vi "test_psmc.vi"() -> ()   [LabVIEW 2014]
uses:
  <vilib>/Platform/TimedLoop/XDataNode/timing_clust.ctl
  <vilib>/Platform/TimedLoop/XDataNode/nitl_modes.ctl
  <vilib>/Platform/TimedLoop/XDataNode/wakeup.ctl
  <vilib>/platform/TimedLoop/XDataNode/XDataNode.xnode
  <vilib>/Platform/TimedLoop/XDataNode/XDNodeRunTimeDep.lvlib
  <vilib>/ptbypt/NI_PtbyPt.lvlib
panel:
  in  "pd":dbl
  out "M1":T1(graph)={"M1 desired speed"=-0.04979126824650304, "M1 position"=nan}
  in  "stop":bool
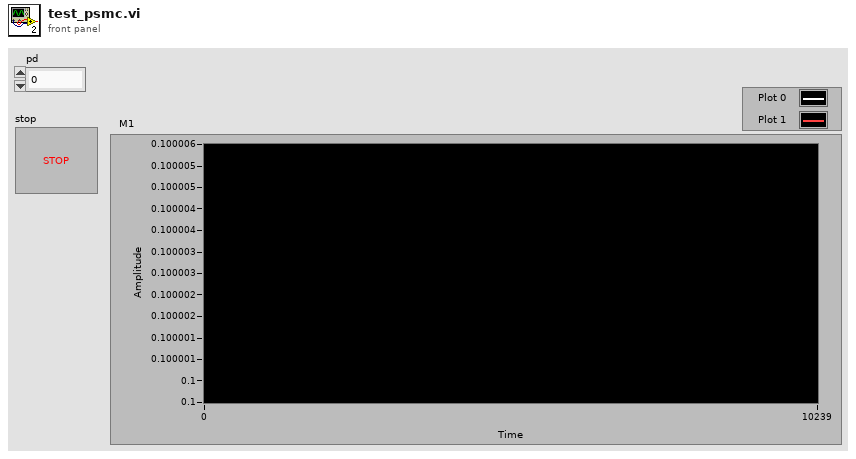
[diagram p1: front panel]
types:
  T1 = cluster{"M1 desired speed":dbl, "M1 position":dbl}
  T2 = typedef "XDNodeRunTimeDep.lvlib/timing_clust.ctl" = cluster{"Expected End [f-1]":u64, "Actual End [f-1]":u64, "Finished Late? [f-1]":bool, "Expected End [i-1]":u64, "Actual End [i-1]":u64, "Finished Late? [i-1]":bool, "Expected Start [i]":u64, "Actual Start [i]":u64, "Expected Start [f]":u64, "Actual Start [f]":u64, "Source Name":string, "Structure Name":string, "Period":i64, "Deadline":i64, "Offset":i64, "Start":i64, "Priority":i32, "Timeout":i32, "Mode":T3, "Wakeup Reason":T4, "Error":errorcluster, "Source Type":string, "Secondary Source Type":string, "Global End Time":u64, "Global Start Time":u64, "Frame Duration":u64, "Iteration Duration":u64, "Assigned CPU":i32, "I/O Scan Engine Mode":u32}
  T3 = typedef "XDNodeRunTimeDep.lvlib/nitl_modes.ctl" = enum32{"No Change", "Process missed periods, maintain original phase", "Discard missed periods, maintain original phase", "Process missed periods, ignore original phase", "Discard missed periods, ignore original phase"}
  T4 = typedef "XDNodeRunTimeDep.lvlib/wakeup.ctl" = enum32{"Normal", "Aborted", "Asynchronous wakeup", "Timing source error", "Timed loop error", "Timeout"}
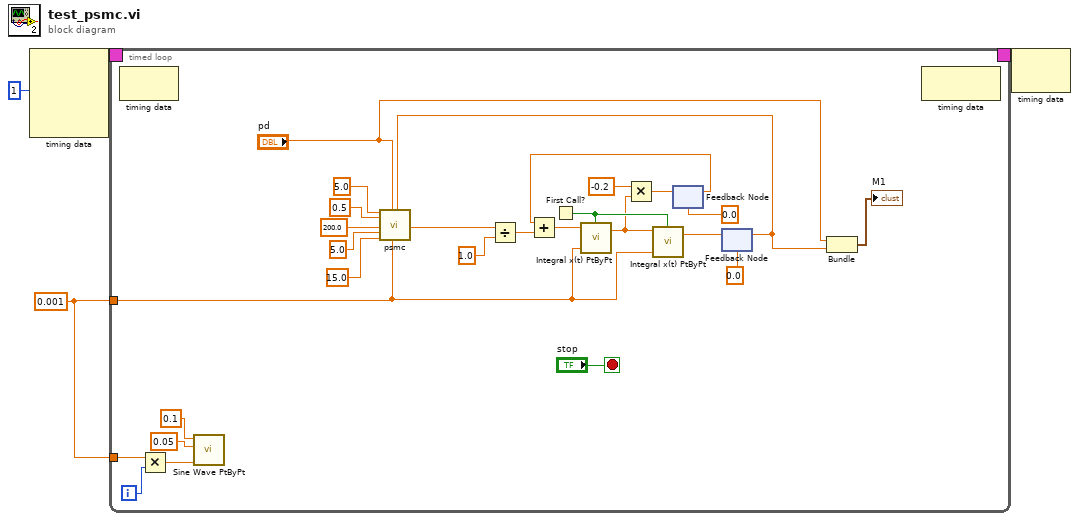
[diagram p0: block diagram]
diagram:
  w1 = 0.001 ("T")
  n1 = node-c288(i64 1 ("Period")) -> (w4:T2)  [unwired: 3 in]
  n2 = timed-loop {
    timing: w4 -> [_]
    timing-out: [_] -> w3
    tunnel: w1 -> [w16]
    tunnel: w1 -> [w15]
    i -> [w17]
    stop <- "stop" stop-if-true
    n3 = node-c288() -> ()  [unwired: 1 in, 1 out]
    n4 = Multiply(x=w16, y=w17) -> (x*y=w20:dbl)
    n5 = call <vilib>:"Sine Wave PtByPt.vi"("time"=w20, "frequency"=0.05, "amplitude"=0.1) -> ()  [unwired: 1 in, 1 out]
    n6 = First Call?() -> (First Call?: T/F=w26:bool)
    n7 = feedback #1(0.0) -> (w22:dbl)
    n8 = feedback #2(0.0 ("integral x(t)")) -> (w9:dbl)
    n9 = call "psmc.vi"("F"=5.0, "H"=0.5, "K"=200.0, "L"=5.0, "B"=15.0, "pd"="pd", "T"=w15, "p"=w9) -> ("f"=w23:dbl)  [unwired: 11 in]
    n10 = Divide(x=w23, y=1.0) -> (x/y=w29:dbl)
    n11 = Add(x=w22, y=w29) -> (x+y=w30:dbl)
    n12 = call <vilib>:"Integral x(t) PtByPt.vi"("initialize"=w26, "dt"=w15, "x"=w30) -> ("integral x(t)"=w25:dbl)  [unwired: 1 in, 1 out]
    n13 = Multiply(x=-0.2, y=w25) -> (x*y=w27:dbl)
    n14 = call <vilib>:"Integral x(t) PtByPt.vi"("initialize"=w26, "dt"=w15, "x"=w25) -> ("integral x(t)"=w21:dbl)  [unwired: 1 in, 1 out]
    n15 = feedback-in #1(w27) -> ()
    n16 = feedback-in #2(w21) -> ()
    n17 = Bundle("pd"="pd", "integral x(t)"=w9) -> (→"M1":cluster{"pd":dbl, "integral x(t)":dbl})  [unwired: 1 in]
    n18 = node-c288() -> ()  [unwired: 1 in, 1 out]
  }
  n19 = node-c288(w3) -> ()  [unwired: 1 out]
